vi "t.vi"() -> ()   [LabVIEW 2014]
uses:
  user.lib/_NEVSTOP/JKI State Machine ++/JKI-State-Machine-Plus.lvlib
panel:
  out "State History":string
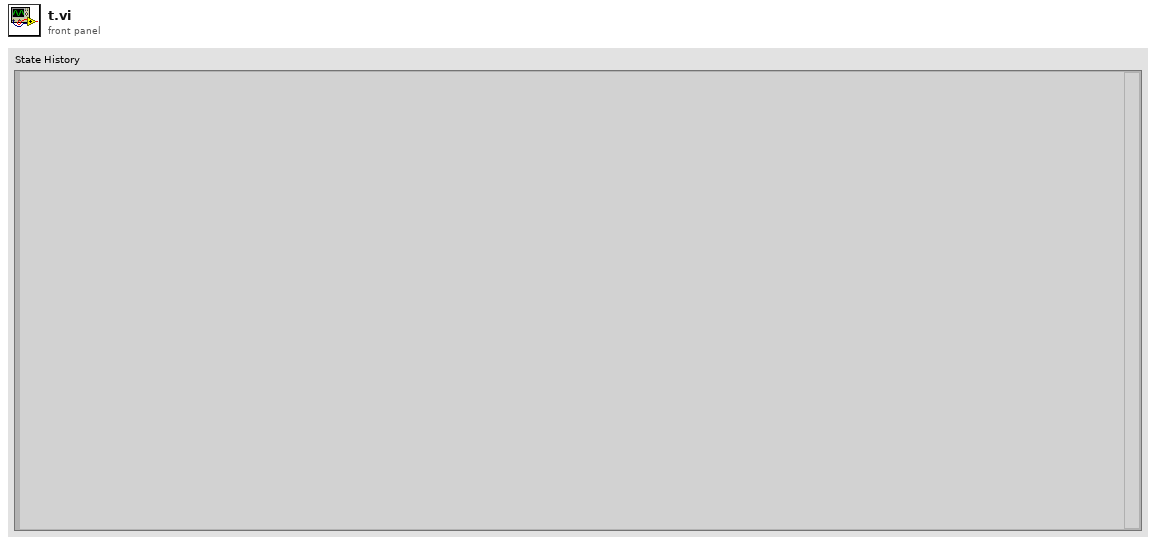
[diagram p1: front panel]
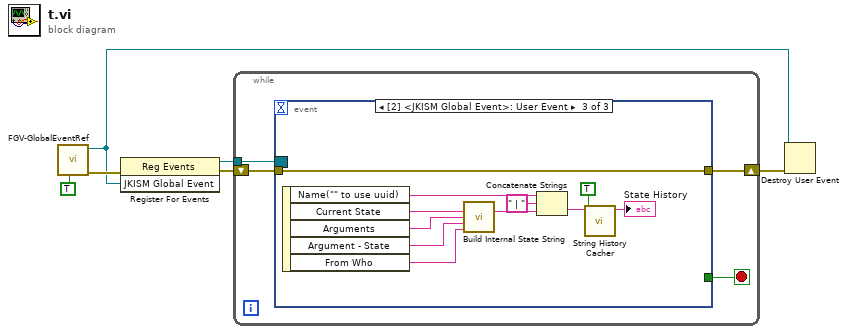
[diagram p0: block diagram]
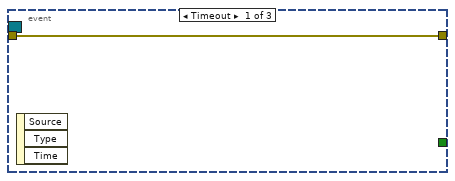
[diagram p2: hidden frame]
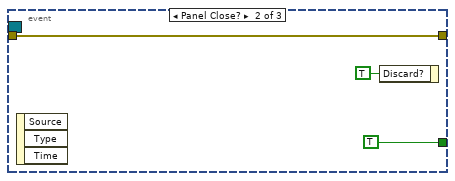
[diagram p3: hidden frame]
diagram:
  n1 = call "FGV-GlobalEventRef.vi"("Create(F)"=TRUE) -> ("error out"=w6:errorcluster, "JKISM Global Event"=w2:refnum<user-event>)  [unwired: 9 in]
  n2 = register-events(error in=w6, w2) -> (reference out=w5:refnum<event-registration>, error out=w4:errorcluster)  [unwired: 1 in]
  n3 = while {
    tunnel: w5 -> [w10]
    shift-right: [w8] -> w3
    shift-left: w4 -> [w9]
    stop <- w7 stop-if-true
    n4 = event shown="[2] <JKISM Global Event>: User Event" {
      selector: w10 -> [_ _ _]
      dyn-events: _ -> [_ _ _]
      timeout: _ -> [_ _ _]
      tunnel: w9 -> [w11 w14 w25]
      tunnel: [w11 w14 w25] -> w8
      tunnel: [_ TRUE ("Discard?") _] -> w7
      event Timeout {
        n5 = event-data() -> ()  [unwired: 1 in, 3 out]
      }
      event Panel Close? {
        n6 = event-data() -> ()  [unwired: 1 in, 3 out]
        n7 = event-data("Discard?"=TRUE) -> ()  [unwired: 1 in, 1 out]
      }
      event User Event {
        n8 = event-data() -> ("Name(\"\" to use uuid)"=w16:string, "Current State"=w21:string, "Arguments"=w20:string, "Argument - State"=w19:string, "From Who"=w18:string)  [unwired: 1 in]
        n9 = call "Build Internal State String.vi"("State"=w21, "Arguments (\"\")"=w20, "Arg-State (\"\")"=w19, "Source (\"\")"=w18) -> ("State with Arguments"=w24:string)  [unwired: 11 in]
        n10 = Concatenate Strings(w16, " | " ("string"), w24) -> (w17:string)
        n11 = call "String History Cacher.vi"("Include Timestamp(F)"=TRUE, "String"=w17) -> ("String Cache"=→"State History":string)  [unwired: 9 in]
      }
    }
  }
  n12 = Destroy User Event(user event=w2, error in=w3) -> ()  [unwired: 1 out]
